vi "Realtime Clock-Dual.vi"() -> ()   [LabVIEW 2009]
uses:
  <vilib>/NXT/Block Support/NXT_InputPort.ctl
  <vilib>/NXT/Subs/LVHSConnector.ctl
  mindsensors.com LVEE Toolkit/Dual/Realtime Clock-DM.vi
panel:
  out "NXT dup":T1={"error"={"status"=FALSE, "code"=0, "source"=""}, "address"="", "NXT #"=-1, "Show Error"=TRUE} caption="NXT"
  in  "NXT":T1={"error"={"status"=FALSE, "code"=0, "source"=""}, "address"="", "NXT #"=-1, "Show Error"=TRUE}
  in  "stop":bool
  out "Month":dbl
  out "Minute":dbl
  out "Year":dbl
  out "Hour":dbl
  out "Date":dbl
  out "Second":dbl
  out "date string":string
  out "time string":string
  in  "Input Port":T2 items=["Port 1", "Port 2", "Port 3", "Port 4"]
  # "mindsensors.com\nCopyright (c) 2009 by mindsensors.com\nEmail: info (<at>) mindsensors (<dot>) com\n\nThis program is free software. You can redistribute it and/or modify\nit under the terms of the GNU General Public License as published by\nthe Free Software Foundation; version 3 of the License.\nRead the license at: http://www.gnu.org/licenses/gpl.txt"
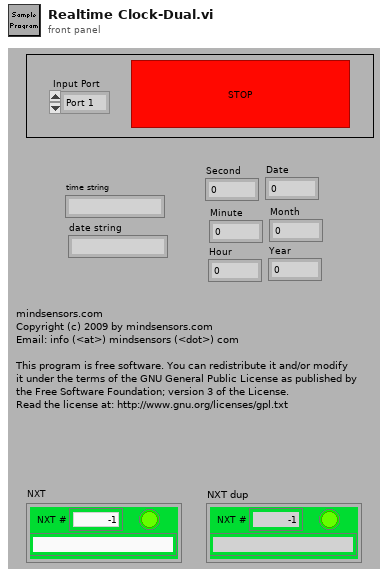
[diagram p1: front panel]
types:
  T1 = typedef "LVHSConnector.ctl" = cluster{"error":errorcluster, "address":string, "NXT #":i32, "Show Error":bool}
  T2 = typedef "NXT_InputPort.ctl" = u8
  T3 = cluster{"date string":string, "date":i8, "month":i8, i16, "time string":string, "Hour":i8, "minute":i8, "second":i8}
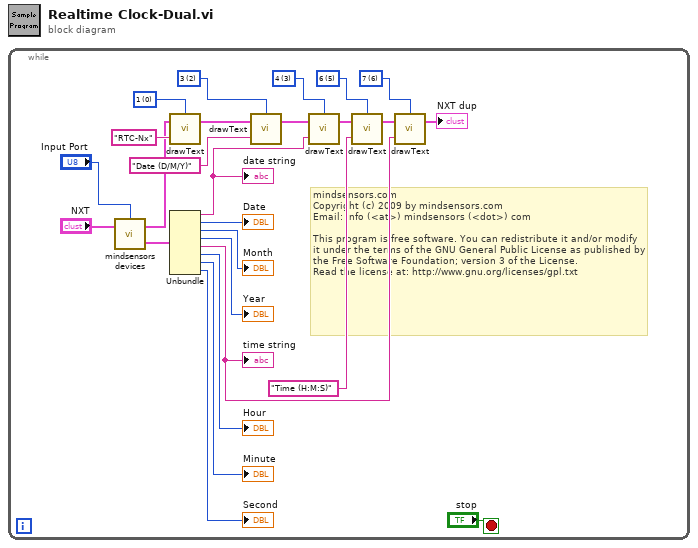
[diagram p0: block diagram]
diagram:
  n1 = while {
    stop <- "stop" stop-if-true
    w11 = i16 0 items=["1", "2", "3", "4", "5", "6", "7", "8"] ("Line")
    w13 = i16 5 items=["1", "2", "3", "4", "5", "6", "7", "8"] ("Line")
    w15 = i16 2 items=["1", "2", "3", "4", "5", "6", "7", "8"] ("Line")
    w16 = i16 3 items=["1", "2", "3", "4", "5", "6", "7", "8"] ("Line")
    w17 = i16 6 items=["1", "2", "3", "4", "5", "6", "7", "8"] ("Line")
    # "mindsensors.com\nCopyright (c) 2009 by mindsensors.com\nEmail: info (<at>) mindsensors (<dot>) com\n\nThis program is free software. You can redistribute it and/or modify\nit under the terms of the GNU General Public License as published by\nthe Free Software Foundation; version 3 of the License.\nRead the license at: http://www.gnu.org/licenses/gpl.txt"
    n2 = call-poly "mindsensors devices.vi"("NXT"="NXT", "Input Port"="Input Port") -> ("Output of Realtime Clock"=w1:T3, "NXT dup"=w7:T1)  [unwired: 1 in]
    n3 = call <vilib>:"drawText.vi"("Text"="RTC-Nx", "NXT"=w7, "Line"=w11) -> ("NXT"=w6:T1)  [unwired: 1 in]
    n4 = Unbundle(w1) -> ("date string"=w9:string, "date"=→"Date":i8, "month"=→"Month":i8, →"Year":i16, "time string"=w8:string, "Hour"=→"Hour":i8, "minute"=→"Minute":i8, "second"=→"Second":i8)
    "time string" <- w8
    "date string" <- w9
    n5 = call <vilib>:"drawText.vi"("Text"="Date (D/M/Y)", "NXT"=w6, "Line"=w15) -> ("NXT"=w5:T1)  [unwired: 1 in]
    n6 = call <vilib>:"drawText.vi"("Text"=w9, "NXT"=w5, "Line"=w16) -> ("NXT"=w4:T1)  [unwired: 1 in]
    n7 = call <vilib>:"drawText.vi"("Text"="Time (H:M:S)", "NXT"=w4, "Line"=w13) -> ("NXT"=w3:T1)  [unwired: 1 in]
    n8 = call <vilib>:"drawText.vi"("Text"=w8, "NXT"=w3, "Line"=w17) -> ("NXT"=→"NXT dup":T1)  [unwired: 1 in]
  }
